vi "DAQmx Create Channel (TEDS-AI-Sound Pressure-Microphone).vi"(0 "task in":refnum<k21>, 1 "maximum sound pressure level":dbl=100.0 format="%0.2f", 3 "input terminal configuration":i32(ring)=-1 items=["default"=-1, "RSE"=10083, "NRSE"=10078, "Differential"=10106, "Pseudodifferential"=12529], 5 "physical channels":tag, 6 "current excitation source":i32(ring)=10200 items=["Internal"=10200, "External"=10167, "None"=10230], 7 "name to assign":string, 8 "current excitation value":dbl=0.004, 9 "units":i32(ring)=10081 items=["Pascals"=10081, "From Custom Scale"=10065], 11 "error in":errorcluster, 12 "custom scale name":tag) -> (4 "task out":refnum<k21>, 15 "error out":errorcluster)   [LabVIEW 2013]
doc: "Creates channel(s) that use a microphone to measure sound pressure. You must configure the physical channel(s) with TEDS information to use this VI."
uses:
  C:/Program Files/National Instruments/LabVIEW 2013/resource/objmgr/daqmx.rc
panel:
  # "input limits"
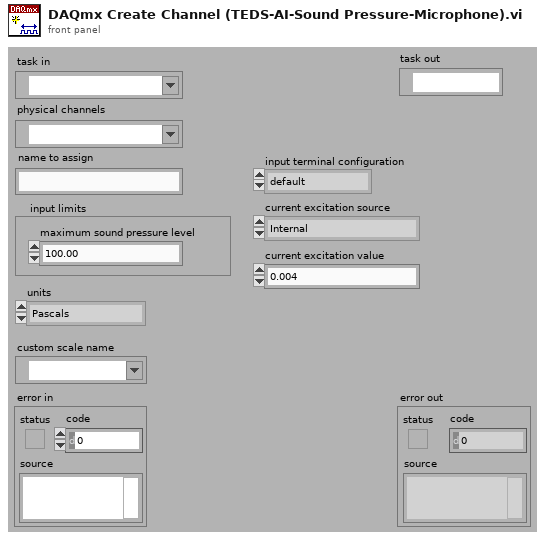
[diagram p1: front panel]
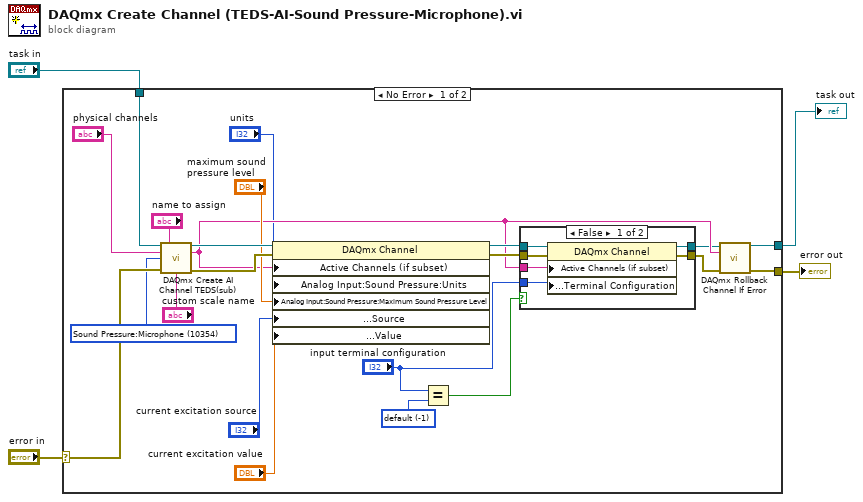
[diagram p0: block diagram]
diagram:
  n1 = case shown="No Error" "error in" {
    selector: "error in" -> [w24 w36]
    tunnel: [w18 w36] -> w2
    tunnel: "task in" -> [w25 w35]
    tunnel: [w19 w35] -> w1
    frame No Error {
      w13 = -1 items=["default"=-1, "differential"=10106, "RSE"=10083, "NRSE"=10078] ("input terminal configuration")
      w15 = 10354 items=["Voltage"=10322, "Current"=10134, "More:Voltage:Custom with Excitation"=10323, "More:Current:Custom with Excitation"=10136, "Frequency"=10181, "Period"=10257, "Resistance"=10278, "Temperature:Thermocouple"=10303, "Temperature:Thermistor"=10302, "Temperature:RTD"=10301, "Temperature:Built-in Sensor"=10311, "Strain Gage"=10300, "LVDT"=10352, "RVDT"=10353, "Accelerometer:Voltage Input"=10355, "Accelerometer:Current Input"=10356, "Sound Pressure:Microphone"=10354] ("measurement type")
      n2 = call "DAQmx Create AI Channel TEDS(sub).vi"("task in"=w25, "virtual channel name"="name to assign", "physical channel name"="physical channels", "measurement type"=w15, "error in"=w24, "custom scale"="custom scale name") -> ("task out"=w26:refnum<k21>, "channel names"=w10:string, "error out"=w21:errorcluster)  [unwired: 7 out]
      n3 = property class="DAQmx Channel"(reference=w26, error in=w21, "Active Channels (if subset)"=w10, "Analog Input:Sound Pressure:Units"="units", "Analog Input:Sound Pressure:Maximum Sound Pressure Level"="maximum sound pressure level", "Analog Input:General Properties:Signal Conditioning:Excitation:Source"="current excitation source", "Analog Input:General Properties:Signal Conditioning:Excitation:Value"="current excitation value") -> (reference out=w12:refnum<k21>, error out=w11:errorcluster)
      n4 = Equal?(x="input terminal configuration", y=w13) -> (x = y?=w8:bool)
      n5 = case shown="False" w8 {
        tunnel: w11 -> [w32 w34]
        tunnel: [w31 w33] -> w7
        tunnel: [w30 w34] -> w6
        tunnel: "input terminal configuration" -> [w29 _]
        tunnel: w10 -> [w28 _]
        tunnel: w12 -> [w27 w33]
        frame False {
          n6 = property class="DAQmx Channel"(reference=w27, error in=w32, "Active Channels (if subset)"=w28, "Analog Input:General Properties:Input Configuration:Terminal Configuration"=w29) -> (reference out=w31:refnum<k21>, error out=w30:errorcluster)
        }
        frame True {
        }
      }
      n7 = call "DAQmx Rollback Channel If Error.vi"("task in"=w7, "channel names"=w10, "error in"=w6) -> ("task out"=w19:refnum<k21>, "error out"=w18:errorcluster)  [unwired: 11 out]
    }
    frame Error {
    }
  }
  "error out" <- w2
  "task out" <- w1
